vi "Day 11-2.vi"() -> ()   [LabVIEW 2020]
uses:
  <vilib>/regexp/Match Regular Expression.xnode
panel:
  out "Answer":i32
  out "Array":i32[][](array[numeric])
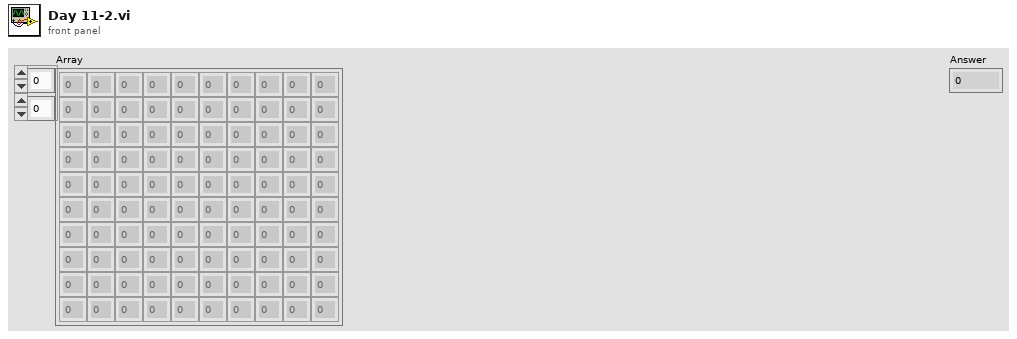
[diagram p1: front panel]
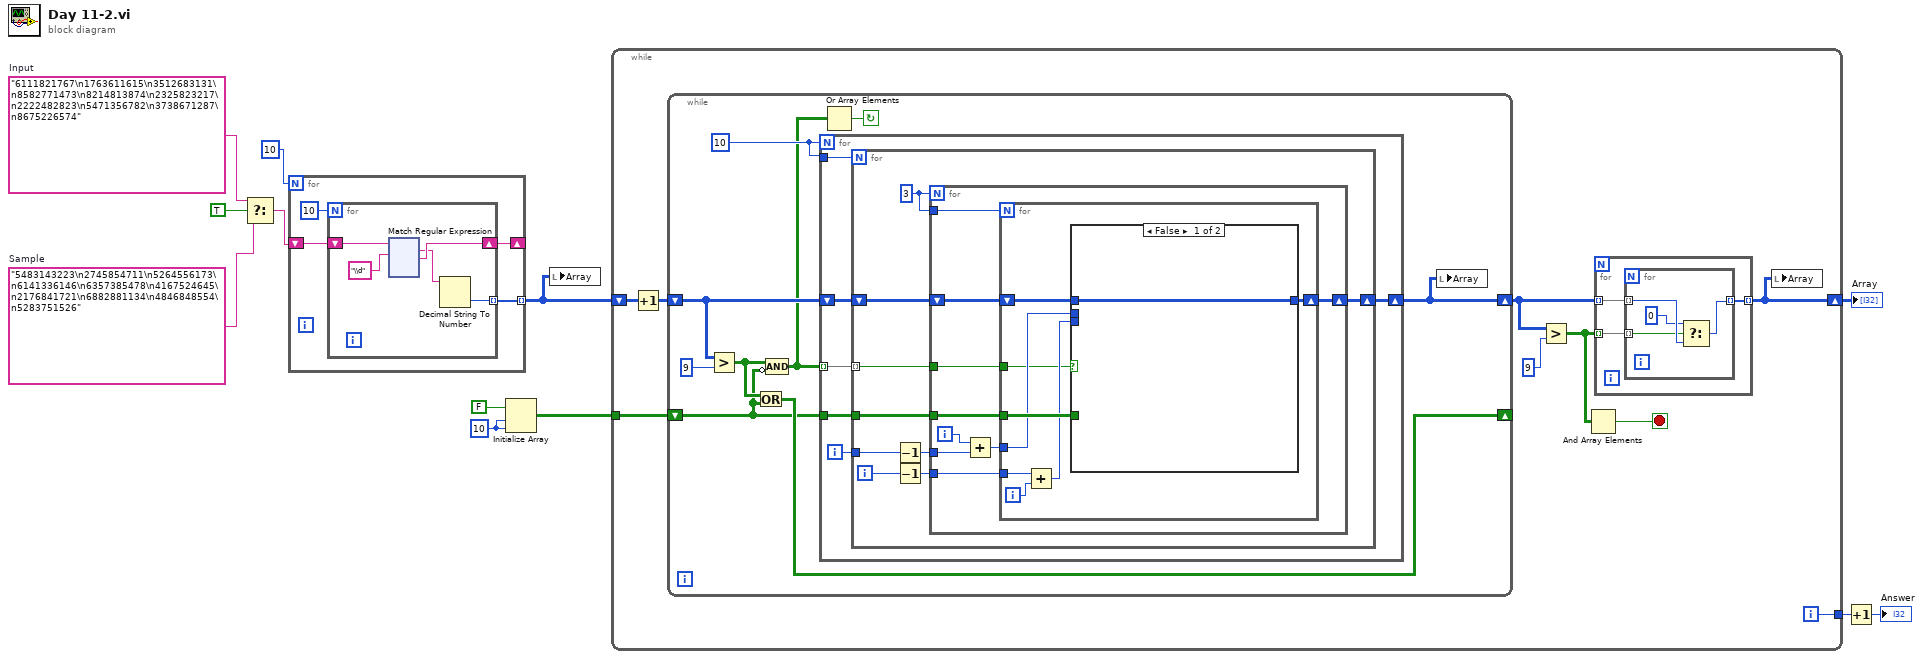
[diagram p0: block diagram]
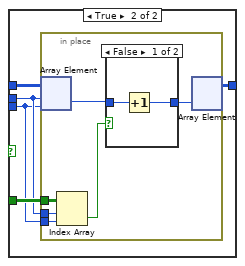
[diagram p2: hidden frame]
diagram:
  w6 = 10 ("dimension size")
  w10 = "5483143223\n2745854711\n5264556173\n6141336146\n6357385478\n4167524645\n2176841721\n6882881134\n4846848554\n5283751526"  # Sample
  w11 = "6111821767\n1763611615\n3512683131\n8582771473\n8214813874\n2325823217\n2222482823\n5471356782\n3738671287\n8675226574"  # Input
  n1 = Select(t=w11, s=TRUE, f=w10) -> (s? t:f=w9:string)
  n2 = for {
    N: 10 -> [_]
    shift-right: [w15] -> _
    shift-left: w9 -> [w16]
    tunnel: [w13] -> w3 mode=indexing
    n3 = for {
      N: 10 -> [_]
      shift-right: [w19] -> w15
      shift-left: w16 -> [w21]
      tunnel: [w17] -> w13 mode=indexing
      n4 = xnode "Match Regular Expression"("input string"=w21, "regular expression"="\\d") -> ("whole match"=w18:string, "after match"=w19:string)  [unwired: 4 in, 3 out]
      n5 = Decimal String To Number(string=w18) -> (number=w17:i32)  [unwired: 2 in, 1 out]
    }
  }
  n6 = Initialize Array(FALSE, w6, w6) -> (w4:bool[][])
  n7 = local write "Array"(w3) -> ()
  n8 = while {
    shift-right: [w139] -> w7
    shift-left: w3 -> [w144]
    tunnel: w4 -> [w142]
    tunnel: [w136] -> w2
    i -> [w136]
    stop <- w137 stop-if-true
    n9 = Increment(x=w144) -> (x+1=w143:i32[][])
    n10 = while {
      shift-right: [w146] -> w140
      shift-left: w143 -> [w151]
      shift-right: [w149] -> _
      shift-left: w142 -> [w147]
      stop <- w152 continue-if-true
      w150 = 10
      n11 = Greater?(x=w151, y=9) -> (0:w148:bool[][])
      n12 = Or(x=w148, y=w147) -> (x .or. y?=w149:bool[][])
      n13 = Compound Arithmetic op=AND(w148, invert w147) -> (w145:bool[][])
      n14 = for {
        N: w150 -> [_]
        shift-right: [w157] -> w146
        shift-left: w151 -> [w159]
        tunnel: w145 -> [w158] mode=indexing
        tunnel: w150 -> [w155]
        tunnel: w147 -> [w154]
        i -> [w156]
        n15 = for {
          N: w155 -> [_]
          shift-right: [w168] -> w157
          shift-left: w159 -> [w161]
          tunnel: w156 -> [w167]
          tunnel: w158 -> [w160] mode=indexing
          tunnel: w154 -> [w165]
          i -> [w166]
          w162 = 3
          n16 = Decrement(x=w167) -> (x-1=w164:i32)
          n17 = Decrement(x=w166) -> (x-1=w163:i32)
          n18 = for {
            N: w162 -> [_]
            shift-right: [w176] -> w168
            shift-left: w161 -> [w177]
            tunnel: w164 -> [w175]
            tunnel: w163 -> [w174]
            tunnel: w165 -> [w172]
            tunnel: w162 -> [w171]
            tunnel: w160 -> [w169]
            i -> [w170]
            n19 = Add(x=w170, y=w175) -> (x+y=w173:i32)
            n20 = for {
              N: w171 -> [_]
              shift-right: [w183] -> w176
              shift-left: w177 -> [w184]
              tunnel: w173 -> [w181]
              tunnel: w174 -> [w185]
              tunnel: w172 -> [w182]
              tunnel: w169 -> [w178]
              i -> [w179]
              n21 = Add(x=w185, y=w179) -> (x+y=w180:i32)
              n22 = case shown="False" w178 {
                tunnel: w184 -> [w186 w191]
                tunnel: [w186 w190] -> w183
                tunnel: w182 -> [_ w189]
                tunnel: w181 -> [_ w188]
                tunnel: w180 -> [_ w187]
                frame False {
                }
                frame True {
                  n23 = in-place {
                    in-place-border: w189 -> [w195]
                    in-place-border: w188 -> [w194]
                    in-place-border: w187 -> [w193]
                    n24 = in-place-array #1(w191, w188, w187) -> (w197:i32)
                    n25 = Index Array(array=w195, index (row)=w194, index (col)=w193) -> (element=w192:bool)
                    n26 = case shown="False" w192 {
                      tunnel: w197 -> [w199 w200]
                      tunnel: [w198 w200] -> w196
                      frame False {
                        n27 = Increment(x=w199) -> (x+1=w198:i32)
                      }
                      frame True {
                      }
                    }
                    n28 = in-place-array #1(w196) -> (w190:i32[][])  [unwired: 2 out]
                  }
                }
              }
            }
          }
        }
      }
      n29 = Or Array Elements(Boolean array=w145) -> (logical OR=w152:bool)
      n30 = local write "Array"(w146) -> ()
    }
    n31 = Greater?(x=w140, y=9) -> (0:w138:bool[][])
    n32 = And Array Elements(Boolean array=w138) -> (logical AND=w137:bool)
    n33 = for {
      tunnel: w140 -> [w203] mode=indexing
      tunnel: w138 -> [w202] mode=indexing
      tunnel: [w201] -> w139 mode=indexing
      n34 = for {
        tunnel: w203 -> [w207] mode=indexing
        tunnel: w202 -> [w205] mode=indexing
        tunnel: [w204] -> w201 mode=indexing
        n35 = Select(t=0, s=w205, f=w207) -> (s? t:f=w204:i32)
      }
    }
    n36 = local write "Array"(w139) -> ()
  }
  "Array" <- w7
  n37 = Increment(x=w2) -> (x+1=→"Answer":i32)
